vi "Read Accelerometer Range.vi"(8 "error in (no error)":errorcluster, 11 "LSM9DS1 IMU in":refnum<class "LSM9DS1 IMU.lvclass">) -> (0 "error out":errorcluster, 2 "Accelerometer Range":T1, 3 "LSM9DS1 IMU out":refnum<class "LSM9DS1 IMU.lvclass">)   [LabVIEW 2020, in "LSM9DS1 IMU.lvclass"]
uses:
  LSM9DS1 IMU.lvclass
  Accelerometer Range.ctl
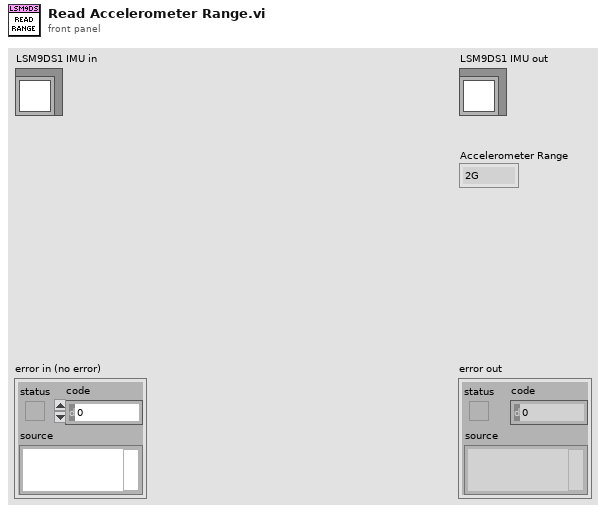
[diagram p1: front panel]
types:
  T1 = typedef "LSM9DS1 IMU.lvclass/Accelerometer Range.ctl" = enum16{"2G", "4G", "8G", "16G"}
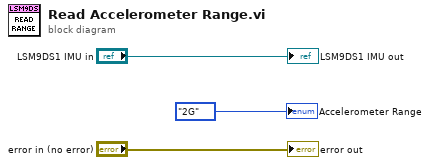
[diagram p0: block diagram]
diagram:
  "error out" <- "error in (no error)"
  "LSM9DS1 IMU out" <- "LSM9DS1 IMU in"
  "Accelerometer Range" <- Accelerometer_Range."2G" ("Accelerometer Range")
